vi "Set Multiple Instances Mode.vi"(7 "Allow multiple instances? (True)":bool=TRUE, 8 "error in (no error)":errorcluster, 11 "configuration file path":path) -> (0 "error out":errorcluster)   [LabVIEW 2020]
doc: "Adds 'allowmultipleinstances' key to ini file."
uses:
  <vilib>/Utility/config.llb/NI_LVConfig.lvlib
  <vilib>/Utility/config.llb/Write Key (Boolean).vi
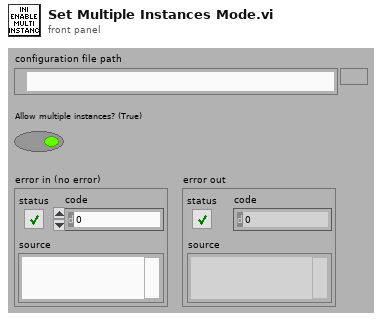
[diagram p1: front panel]
types:
  T1 = typedef "NI_LVConfig.lvlib/Config Data RefNum.ctl" = refnum<k1>
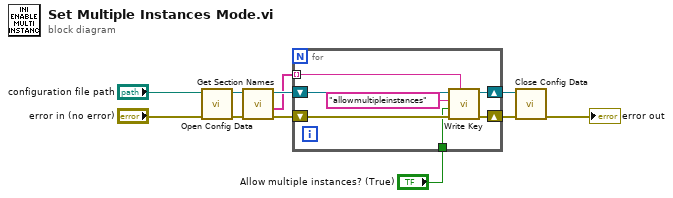
[diagram p0: block diagram]
diagram:
  n1 = call <vilib>:"Open Config Data.vi"("error in (no error)"="error in (no error)", "configuration file path"="configuration file path") -> ("error out"=w8:errorcluster, "refnum"=w7:T1)  [unwired: 7 in, 1 out]
  n2 = call <vilib>:"Get Section Names.vi"("error in (no error)"=w8, "refnum"=w7) -> ("error out"=w11:errorcluster, "section names"=w3:string[], "refnum out"=w10:T1)  [unwired: 7 in]
  n3 = for {
    shift-right: [w16] -> w6
    shift-left: w11 -> [w18]
    shift-right: [w15] -> w4
    shift-left: w10 -> [w17]
    tunnel: w3 -> [w14] mode=indexing
    tunnel: "Allow multiple instances? (True)" -> [w12]
    n4 = call-poly <vilib>:"Write Key.vi"("section"=w14, "error in (no error)"=w18, "value"=w12, "key"="allowmultipleinstances", "refnum"=w17) -> ("error out"=w16:errorcluster, "refnum out"=w15:T1)  [unwired: 4 in, 1 out]
  }
  n5 = call <vilib>:"Close Config Data.vi"("error in (no error)"=w6, "refnum"=w4) -> ("error out"=→"error out":errorcluster)  [unwired: 8 in, 1 out]
